vi "ReadImageFile.vi"(6 "Use File Path Image Type":bool=TRUE, 7 "File Path":path, 8 "error in":errorcluster, 9 "ImageFileOptions":T1 {"File Data Type" items=["1 bit", "2 bits", "4 bits", "8 bits", "16 bits (unsigned)", "16 bits (signed)", "16 bits (RGB chunky)", "24 bits (RGB chunky)", "24 bits (RGB planar)", "32 bits (unsigned)", "32 bits (signed)", "32 bits (RGB chunky)", "32 bits (float)", "48 bits (Complex 2x24 int)", "64 bits (Complex 2x32 float)", "32 bits (HSL)"]; "Read Raw File" items=["Don't Read Raw File ", "Read Raw File"]}, 10 "Load Color Pallete":bool, 11 "Image Reference In":T4) -> (0 "error out":errorcluster, 1 "Pixel Size":i32, 2 "File Data Type":string, 3 "Image Reference Out":T4, 5 "Color Palette":T3[](array[typedef]))   [LabVIEW 2024, in "OpenLvVision_Image.lvlib" / "File.lvlib"]
doc: "Reads an image from a file (supporting BMP, TIFF, JPEG, JPEG2000, PNG) and can also read non-standard formats if the \"read raw file\" option is enabled."
uses:
  File.lvlib
  Management/TypeDef/Image.ctl
  TypeDef/ColorPaletteValue.ctl
  TypeDef/ImageFileOptions.ctl
  TypeDef/FileDataType.ctl
  Management/Management.lvlib
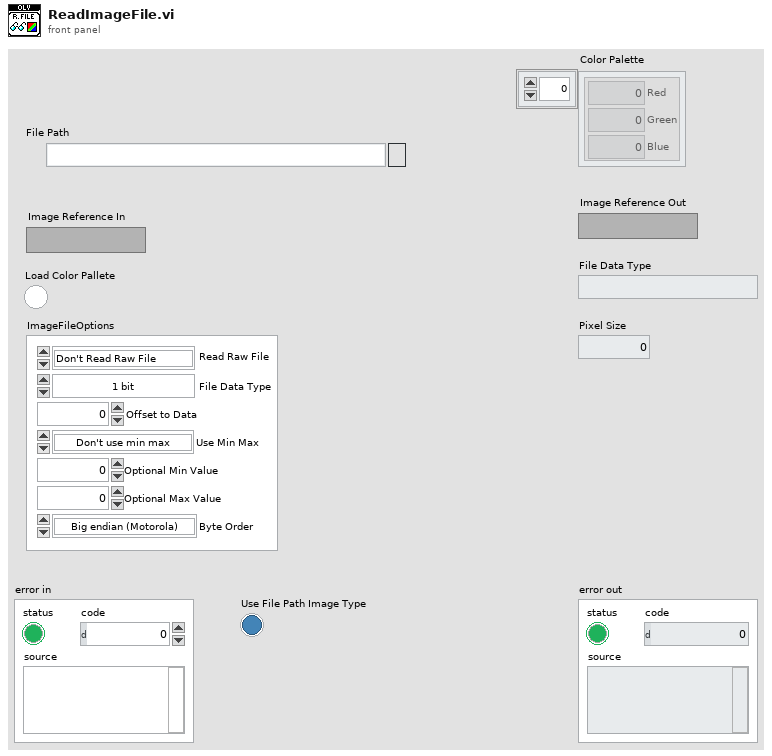
[diagram p1: front panel]
types:
  T1 = typedef "OpenLvVision_Image.lvlib/File.lvlib/ImageFileOptions.ctl" = cluster{"File Data Type":T2, "Offset to Data":i32, "Use Min Max":enum32{"Don't use min max", "Use file values", "Use optional values"}, "Optional Min Value":sgl, "Optional Max Value":sgl, "Byte Order":enum32{"Big endian (Motorola)", "Little endian (Intel)"}, "Read Raw File":i32}
  T2 = typedef "OpenLvVision_Image.lvlib/File.lvlib/FileDataType.ctl" = u32
  T3 = typedef "OpenLvVision_Image.lvlib/File.lvlib/ColorPaletteValue.ctl" = cluster{"Red":u8, "Green":u8, "Blue":u8}
  T4 = typedef "OpenLvVision_Image.lvlib/Management.lvlib/Image.ctl" = refnum<image>
  T5 = typedef "IMAQ Image.ctl" = refnum<image>
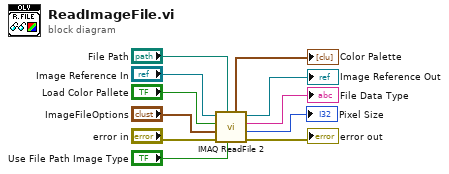
[diagram p0: block diagram]
diagram:
  n1 = call "IMAQ ReadFile 2"("Use File Path Image Type"="Use File Path Image Type", "File Path"="File Path", "error in (no error)"="error in", "File Options"="ImageFileOptions", "Load Color Palette? (No)"="Load Color Pallete", "Image"="Image Reference In") -> ("error out"=→"error out":errorcluster, "File Data Type out"=→"Pixel Size":i32, "File Type out"=→"File Data Type":string, "Image Out"=→"Image Reference Out":T5, "Color Palette out"=→"Color Palette":cluster{"Red":u8, "Green":u8, "Blue":u8}[])  [unwired: 1 in]
